vi "SlackAPI-users.info.vi"(0 "token":string, 7 "user":string, 11 "error in (no error)":errorcluster) -> (6 "user":T1, 10 "is_bot":bool, 15 "error out":errorcluster)   [LabVIEW 2020]
uses:
  Typedefs/Slack-User.ctl
  <vilib>/httpClient/POSTBuffer.vi
  <vilib>/httpClient/LabVIEWHTTPClient.lvlib
panel:
  out "body":string
  out "headers":string
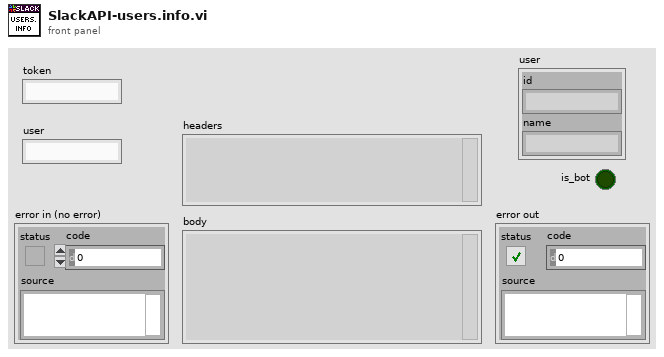
[diagram p1: front panel]
types:
  T1 = typedef "Slack-User.ctl" = cluster{"id":string, "name":string}
  T2 = cluster{"user":cluster{"id":string, "profile":cluster{"real_name":string, "display_name":string}, "is_bot":bool}}
  T3 = typedef "LabVIEWHTTPClient.lvlib/ClientHandle.ctl" = refnum<k1>
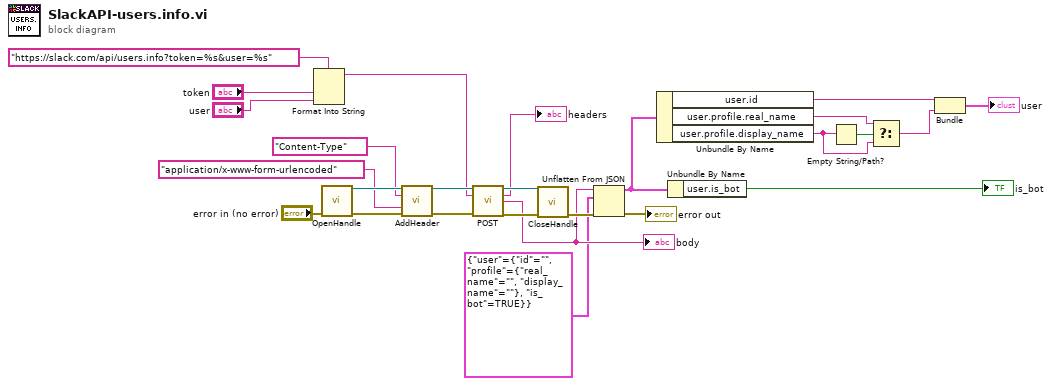
[diagram p0: block diagram]
diagram:
  n1 = Format Into String(format string="https://slack.com/api/users.info?token=%s&user=%s", "token", "user") -> (resulting string=w19:string)  [unwired: 2 in, 1 out]
  n2 = call <vilib>:"OpenHandle.vi"("error in (no error)"="error in (no error)") -> ("client handle out"=w25:T3, "error out"=w26:errorcluster)  [unwired: 13 in]
  n3 = call <vilib>:"AddHeader.vi"("client handle"=w25, "header"="Content-Type", "value"="application/x-www-form-urlencoded", "error in (no error)"=w26) -> ("client handle out"=w21:T3, "error out"=w22:errorcluster)  [unwired: 10 in]
  n4 = call-poly <vilib>:"POST.vi"("client handle"=w21, "url"=w19, "error in (no error)"=w22) -> ("client handle out"=w18:T3, "headers"=→"headers":string, "body"=w11:string, "error out"=w17:errorcluster)  [unwired: 9 in]
  "body" <- w11
  n5 = call <vilib>:"CloseHandle.vi"("client handle"=w18, "error in (no error)"=w17) -> ("error out"=w13:errorcluster)  [unwired: 13 in]
  n6 = Unflatten From JSON(JSON string=w11, type and defaults=T2 {"user"={"id"="", "profile"={"real_name"="", "display_name"=""}, "is_bot"=TRUE}}, error in (no error)=w13) -> (value=w6:T2, error out=→"error out":errorcluster)  [unwired: 4 in]
  n7 = Unbundle By Name(w6) -> ("user.id"=w8:string, "user.profile.real_name"=w3:string, "user.profile.display_name"=w2:string)
  n8 = Unbundle By Name(w6) -> ("user.is_bot"=→"is_bot":bool)
  n9 = Empty String/Path?(string/path=w2) -> (empty?=w4:bool)
  n10 = Select(t=w3, s=w4, f=w2) -> (s? t:f=w1:string)
  n11 = Bundle("id"=w8, "display_name"=w1) -> (→"user":cluster{"id":string, "display_name":string})  [unwired: 1 in]
